vi "Report.vi"(8 "error in":errorcluster, 9 "Received":path, 10 "Approved":path, 11 "Report With Beyond Compare in":refnum<class "Report With Beyond Compare.lvclass">) -> (0 "error out":errorcluster, 2 "Worked?":bool, 3 "Report With Beyond Compare out":refnum<class "Report With Beyond Compare.lvclass">)   [LabVIEW 2020, in "Approval Tests.lvlib" / "Report With Beyond Compare.lvclass"]
uses:
  Report With Beyond Compare.lvclass
  Report With Beyond Compare.lvclass/Report With Beyond Compare.ctl
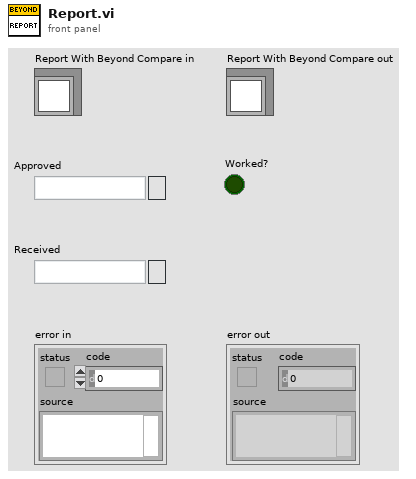
[diagram p1: front panel]
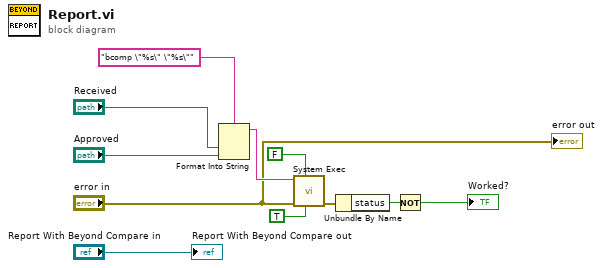
[diagram p0: block diagram]
diagram:
  n1 = Format Into String(format string="bcomp \"%s\" \"%s\"", "Received", "Approved") -> (resulting string=w9:string)  [unwired: 2 in, 1 out]
  n2 = call <vilib>:"System Exec.vi"("run minimized? (F)"=TRUE, "wait until completion? (T)"=FALSE, "error in (no error)"="error in", "command line"=w9) -> ("error out"=w4:errorcluster)  [unwired: 4 in, 3 out]
  n3 = Unbundle By Name(w4) -> ("status"=w2:bool)
  n4 = Not(x=w2) -> (.not. x?=→"Worked?":bool)
  "error out" <- "error in"
  "Report With Beyond Compare out" <- "Report With Beyond Compare in"
